vi "Write Dependencies.vi"(8 "error in (no error)":errorcluster, 10 "Transport":refnum<class "Transport.lvclass">, 11 "SweepControl in":refnum<class "Sweep Control.lvclass">) -> (0 "error out":errorcluster, 3 "SweepControl out":refnum<class "Sweep Control.lvclass">)   [LabVIEW 2019, in "Sweep Control.lvclass"]
uses:
  Sweep Control.lvclass
  <userlib>/LevyLab/Transport/Transport/Transport.lvclass
  Sweep Control.lvclass/Sweep Control.ctl
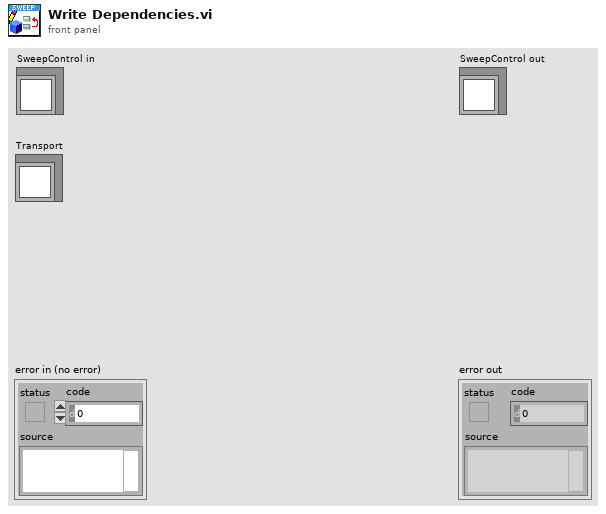
[diagram p1: front panel]
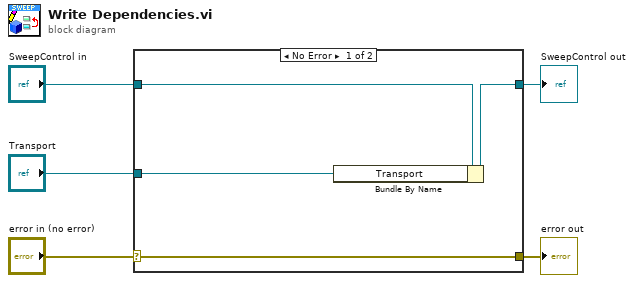
[diagram p0: block diagram]
diagram:
  n1 = case shown="No Error" "error in (no error)" {
    selector: "error in (no error)" -> [w9 w10]
    tunnel: [w9 w10] -> w4
    tunnel: [w7 w11] -> w2
    tunnel: "SweepControl in" -> [w8 w11]
    tunnel: "Transport" -> [w6 _]
    frame No Error {
      n2 = Bundle By Name(cluster=w8, "Transport"=w6) -> (w7:refnum<class "Sweep Control.lvclass">)
    }
    frame Error {
    }
  }
  "error out" <- w4
  "SweepControl out" <- w2
